vi "Stop Global.vi"() -> ()   [LabVIEW 2021]
panel:
  in  "Stop":bool
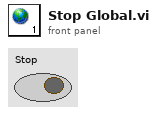
[diagram p1: front panel]
diagram:
